vi "Status Q.vi"(11 "Data Logger Module in":refnum<class "Data Logger DBL Module.lvclass">) -> (2 "Status Q":refnum<class "MessageQ.lvclass">, 3 "Data Logger Module out":refnum<class "Data Logger DBL Module.lvclass">)   [LabVIEW 2020, in "VolatusData.lvlib" / "Data Logger DBL Module.lvclass"]
uses:
  Data Logger DBL Module.lvclass
  Data Logger DBL Module.lvclass/Data Logger DBL Module.ctl
  Volatus/Module/Module.lvclass
  C:/dev/lv20CE/relink/lv-volatus/Volatus/Module/Module.lvclass
  C:/dev/lv20CE/relink/lv-volatus/VolatusData/Data Logger DBL Module/Data Logger DBL Module.lvclass
  Volatus/MessageQ/MessageQ.lvclass
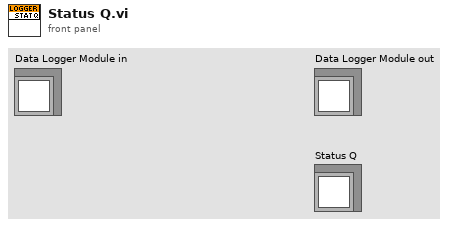
[diagram p1: front panel]
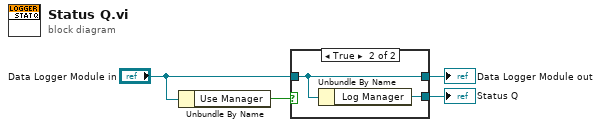
[diagram p0: block diagram]
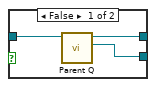
[diagram p2: hidden frame]
diagram:
  n1 = Unbundle By Name("Data Logger Module in") -> ("Use Manager"=w4:bool)
  n2 = case shown="True" w4 {
    tunnel: "Data Logger Module in" -> [w7 w8]
    tunnel: [w5 w9] -> w2
    tunnel: [w6 w8] -> w1
    frame False {
      n3 = call "Parent Q.vi"("Module in"=w7) -> ("Parent Q"=w5:refnum<class "MessageQ.lvclass">, "Module out"=w6:refnum<class "Data Logger DBL Module.lvclass">)  [unwired: 9 in]
    }
    frame True {
      n4 = Unbundle By Name(w8) -> ("Log Manager"=w9:refnum<class "MessageQ.lvclass">)
    }
  }
  "Data Logger Module out" <- w1
  "Status Q" <- w2
